vi "VNA.Read Configuration.vi"(8 "error in (no error)":errorcluster, 11 "VNA":refnum<class "VNA.lvclass">) -> (0 "error out":errorcluster, 2 "Configuration":T1, 3 "VNA out":refnum<class "VNA.lvclass">)   [LabVIEW 2016, in "VNA.lvclass"]
uses:
  VNA.lvclass
  Typedefs/VNA.Configuration--Cluster.ctl
  VNA.lvclass/VNA.ctl
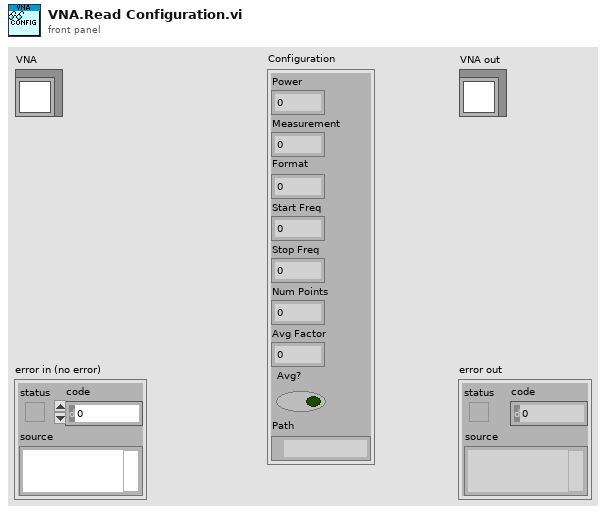
[diagram p1: front panel]
types:
  T1 = typedef "VNA.lvclass/VNA.Configuration--Cluster.ctl" = cluster{"Power":dbl, "Measurement":dbl, "Format":dbl, "Start Freq":dbl, "Stop Freq":dbl, "Num Points":dbl, "Avg Factor":dbl, "Avg?":bool, "Path":path}
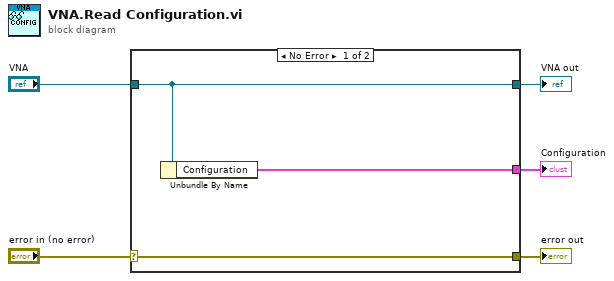
[diagram p0: block diagram]
diagram:
  n1 = case shown="No Error" "error in (no error)" {
    selector: "error in (no error)" -> [w8 w9]
    tunnel: [w8 w9] -> w4
    tunnel: [w7 w10] -> w2
    tunnel: "VNA" -> [w7 w10]
    tunnel: [w6 _] -> w1
    frame No Error {
      n2 = Unbundle By Name(w7) -> ("Configuration"=w6:T1)
    }
    frame Error {
    }
  }
  "error out" <- w4
  "VNA out" <- w2
  "Configuration" <- w1
